vi "工單資訊更新To PLC.vi"(11 "Work No":string caption="工單號碼") -> (0 "error out":errorcluster, 1 "Boolean":bool=TRUE, 2 "NG數":i32, 3 "良品數量":i32)   [LabVIEW 2019]
uses:
  Ctrl/Table Save.ctl
  Ctrl/S1 Station Input.ctl
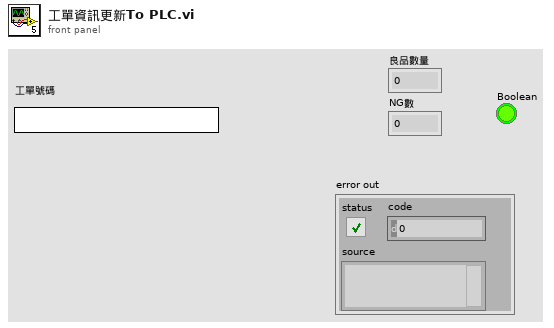
[diagram p1: front panel]
types:
  T1 = typedef "工單號碼_Index.ctl" = enum16{"工單號碼", "產品料號", "品名", "作業員", "生產總數", "量品數量", "NG數量", "良率%"}
  T2 = typedef "Table Save.ctl" = enum16{"initial", "Add", "Write", "Replace", "Delete", "REad", "RedTable", "Load"}
  T3 = typedef "S1 Station Input.ctl" = enum16{"00PLC Alive clock", "01PLC狀態(手動)", "02_備用", "03PC Recipe Change", "04PC→PLC Recipe Save", "05PC→PLC 清線", "06PC ALARM", "07PC首件模式", "08首件PASS", "09工單號碼更換", "10_S0 動作中", "11_S1條碼讀取完成", "12_備用", "13_備用", "14_備用", "15_備用", "16_備用", "17_備用", "18_備用", "19_S0載盤條碼掃描完成"}
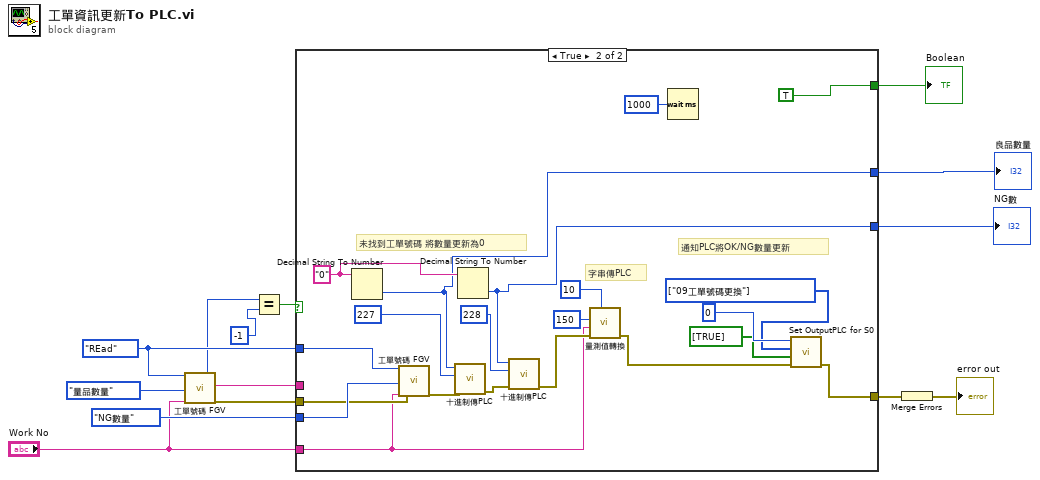
[diagram p0: block diagram]
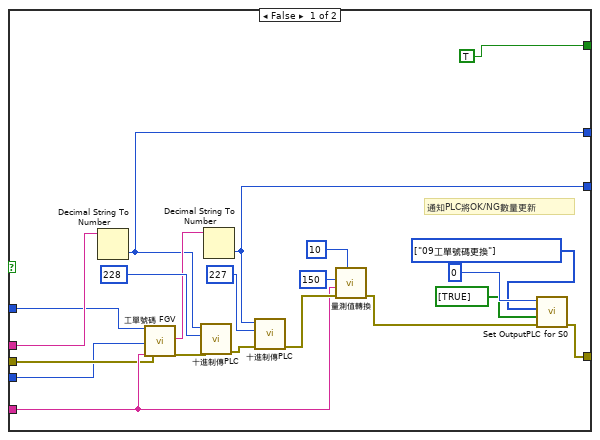
[diagram p2: hidden frame]
diagram:
  w13 = Table_Save."REad" ("Action")
  n1 = call "工單號碼 FGV.vi"("Action"=w13, "工單Data Save Index"=工單號碼_Index."量品數量" ("工單號碼Index"), "工單號碼"="Work No") -> ("工單號碼的Index"=w7:i32, "Read Index Data"=w11:string, "error out"=w10:errorcluster)  [unwired: 9 in, 5 out]
  n2 = Equal?(x=w7, y=-1) -> (x = y?=w6:bool)
  n3 = case shown="True" w6 {
    tunnel: w13 -> [w20 w56]
    tunnel: 工單號碼_Index."NG數量" ("工單號碼Index") -> [w21 w55]
    tunnel: w11 -> [w22 _]
    tunnel: w10 -> [w23 w48]
    tunnel: "Work No" -> [w24 w43]
    tunnel: [w19 w41] -> w5
    tunnel: [w18 w40] -> w3
    tunnel: [w17 w39] -> w2
    tunnel: [TRUE TRUE] -> w1
    frame False {
      w32 = T3[] [enum."09工單號碼更換"] items=["00PLC Alive clock", "01PLC狀態(手動)", "02_備用", "03PC Recipe Change", "04PC→PLC Recipe Save", "05PC→PLC 清線", "06PC ALARM", "07PC首件模式", "08首件PASS", "09工單號碼更換", "10_S0 動作中", "11_S1條碼讀取完成", "12_備用", "13_備用", "14_備用", "15_備用", "16_備用", "17_備用", "18_備用", "19_S0載盤條碼掃描完成"]
      # "通知PLC將OK/NG數量更新"
      n4 = Decimal String To Number(string=w22) -> (number=w18:i32)  [unwired: 2 in, 1 out]
      n5 = call "工單號碼 FGV.vi"("Action"=w20, "工單Data Save Index"=w21, "工單號碼"=w24, "error in (no error)"=w23) -> ("Read Index Data"=w30:string, "error out"=w26:errorcluster)  [unwired: 8 in, 6 out]
      n6 = call "十進制傳PLC.vi"("error in (no error)"=w26, "PLC address"=228, "Input Data"=w18) -> ("error out"=w25:errorcluster)  [unwired: 7 in, 1 out]
      n7 = Decimal String To Number(string=w30) -> (number=w17:i32)  [unwired: 2 in, 1 out]
      n8 = call "十進制傳PLC.vi"("error in (no error)"=w25, "PLC address"=227, "Input Data"=w17) -> ("error out"=w28:errorcluster)  [unwired: 7 in, 1 out]
      n9 = call "量測值轉換.vi"("位數"=10, "error in (no error)"=w28, "input string"=w24, "PLC address"=150) -> ("error out"=w27:errorcluster)  [unwired: 6 in, 1 out]
      n10 = call "Set OutputPLC for S0.vi"("Address In"=0, "Array"=w32, "Sat Coils"=bool[] [TRUE], "error in (no error)"=w27) -> ("Error Out"=w19:errorcluster[])  [unwired: 6 in]
    }
    frame True {
      w42 = "0"
      w51 = T3[] [enum."09工單號碼更換"] items=["00PLC Alive clock", "01PLC狀態(手動)", "02_備用", "03PC Recipe Change", "04PC→PLC Recipe Save", "05PC→PLC 清線", "06PC ALARM", "07PC首件模式", "08首件PASS", "09工單號碼更換", "10_S0 動作中", "11_S1條碼讀取完成", "12_備用", "13_備用", "14_備用", "15_備用", "16_備用", "17_備用", "18_備用", "19_S0載盤條碼掃描完成"]
      # "字串傳PLC"
      # "未找到工單號碼 將數量更新為0"
      # "通知PLC將OK/NG數量更新"
      n11 = Decimal String To Number(string=w42) -> (number=w40:i32)  [unwired: 2 in, 1 out]
      n12 = call "工單號碼 FGV.vi"("Action"=w56, "工單Data Save Index"=w55, "工單號碼"=w43, "error in (no error)"=w48) -> ("error out"=w45:errorcluster)  [unwired: 8 in, 7 out]
      n13 = call "十進制傳PLC.vi"("error in (no error)"=w45, "PLC address"=227, "Input Data"=w40) -> ("error out"=w44:errorcluster)  [unwired: 7 in, 1 out]
      n14 = Decimal String To Number(string=w42) -> (number=w39:i32)  [unwired: 2 in, 1 out]
      n15 = call "十進制傳PLC.vi"("error in (no error)"=w44, "PLC address"=228, "Input Data"=w39) -> ("error out"=w47:errorcluster)  [unwired: 7 in, 1 out]
      n16 = call "量測值轉換.vi"("位數"=10, "error in (no error)"=w47, "input string"=w43, "PLC address"=150) -> ("error out"=w46:errorcluster)  [unwired: 6 in, 1 out]
      n17 = Wait (ms)(milliseconds to wait=u32 1000) -> ()  [unwired: 1 out]
      n18 = call "Set OutputPLC for S0.vi"("Address In"=0, "Array"=w51, "Sat Coils"=bool[] [TRUE], "error in (no error)"=w46) -> ("Error Out"=w41:errorcluster[])  [unwired: 6 in]
    }
  }
  "良品數量" <- w3
  "NG數" <- w2
  "Boolean" <- w1
  n19 = Merge Errors(w5) -> (→"error out":errorcluster)
